vi "adam-4xxxl.vi"() -> ()   [LabVIEW 2024]
panel:
  in  "clear-command":bool
  in  "Channels":T1
  out "concatenated string":string
  in  "Single/Multi Channel":bool
  in  "Deliminator Char":string(combo)
  in  "Manual Command":string="#01"
  out "read buffer":string
  out "Bytes at Port":u32
  in  "send-command":bool
  out "Channel Number":string
  out "Channel State String":string
  out "Device Address":string
  in  "Device Address":i32=1 min=0 max=100 step=1
  in  "baud rate (19200)":u32=19200
  in  "COM Port (COM10)":refnum<visa-resource-name>="COM10"
  in  "Stop Program":bool
  out "command":string
  in  "Channel Number":i32=1 min=0 max=7 step=1
  in  "Channel State Bit":bool
  out "Bytes Written":u32
  out "error":errorcluster
  # "ADAM-4xxx Test VI"
  # "To Use, either:\n- Enter Manual Command in Text box\nOR\n- Set up command using options below\nThen:\n- Press Send Command"
  # "Example Commands:\n  Code   |    Behaviour       | Success | Failed \n---      |---                 |---      |---\nadam-4069 8x Power Relay\n#010000 \t| All Channels: Off  |\t   > \t  | ?AA \n#01000F \t| All Channels: On \t |         |\n#011000 \t| Channel 0: Off \t   |\t        |\n#011001 \t| Channel 0: On \t\t   |         |\n#011100 \t| Channel 1: Off \t\t  |         |\n#011101 \t| Channel 1: On \t    |         |"
  # "adam-4017+ 8x AI\nadam-4018+ 8x T/C & mA\n#01 \t    | All Channels: data |>+data+data...| ?AA \nAA = module address"
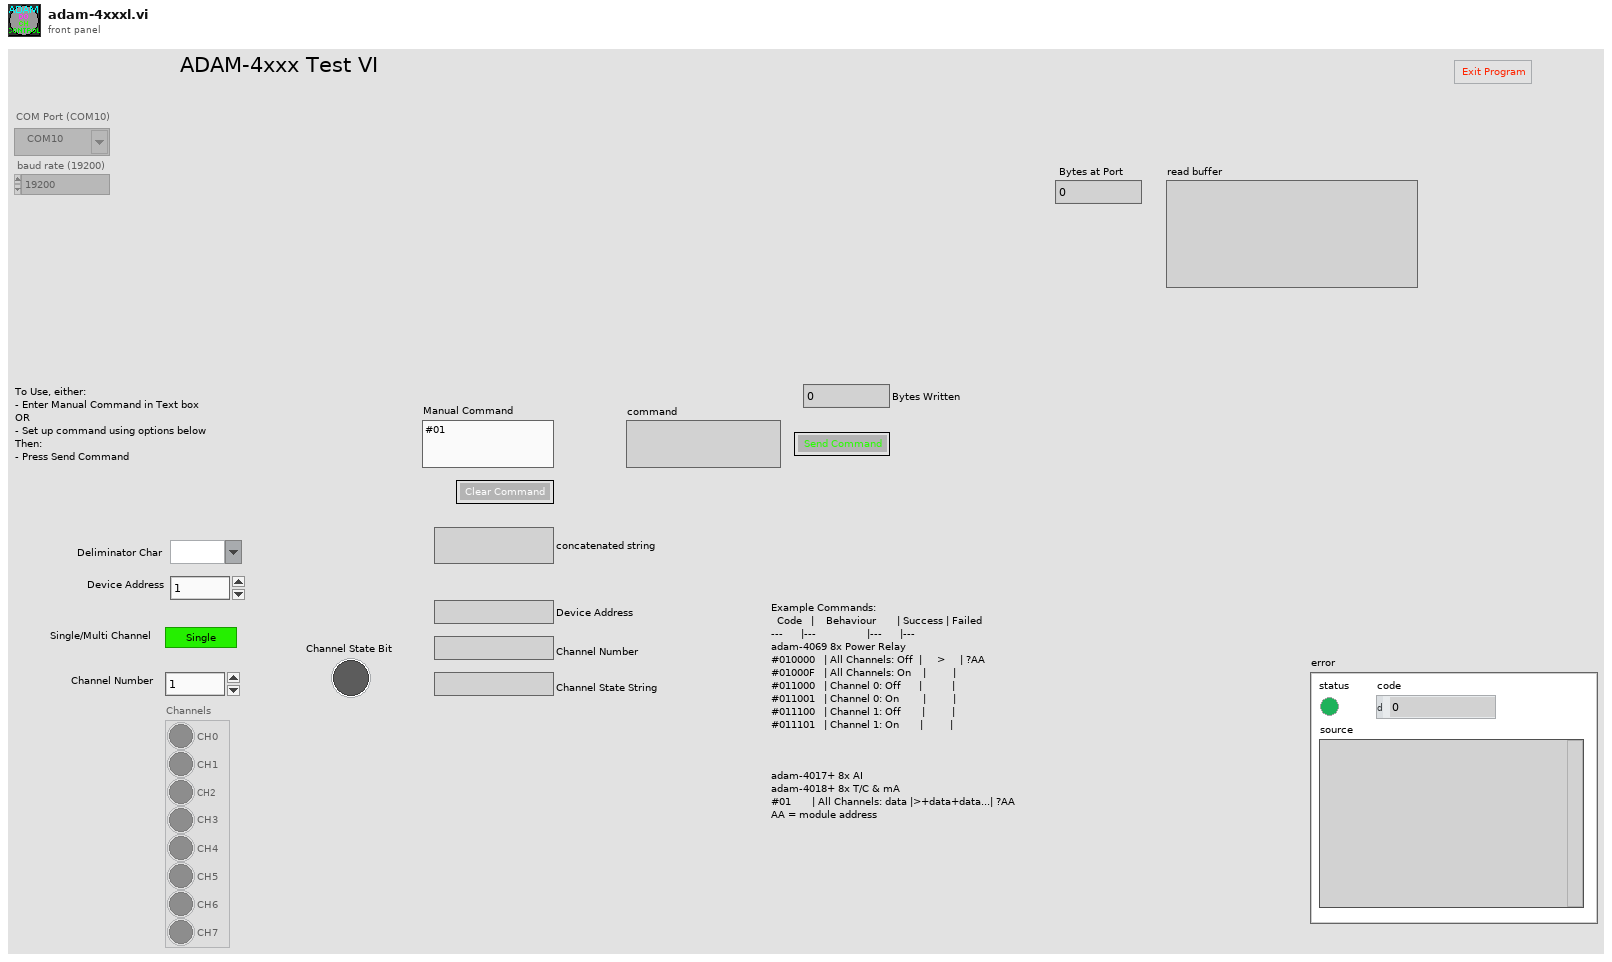
[diagram p1: front panel]
types:
  T1 = cluster{"CH0":bool, "CH1":bool, "CH2":bool, "CH3":bool, "CH4":bool, "CH5":bool, "CH6":bool, "CH7":bool}
  T2 = enum8{"Enabled", "Disabled", "Disabled and Grayed Out"}
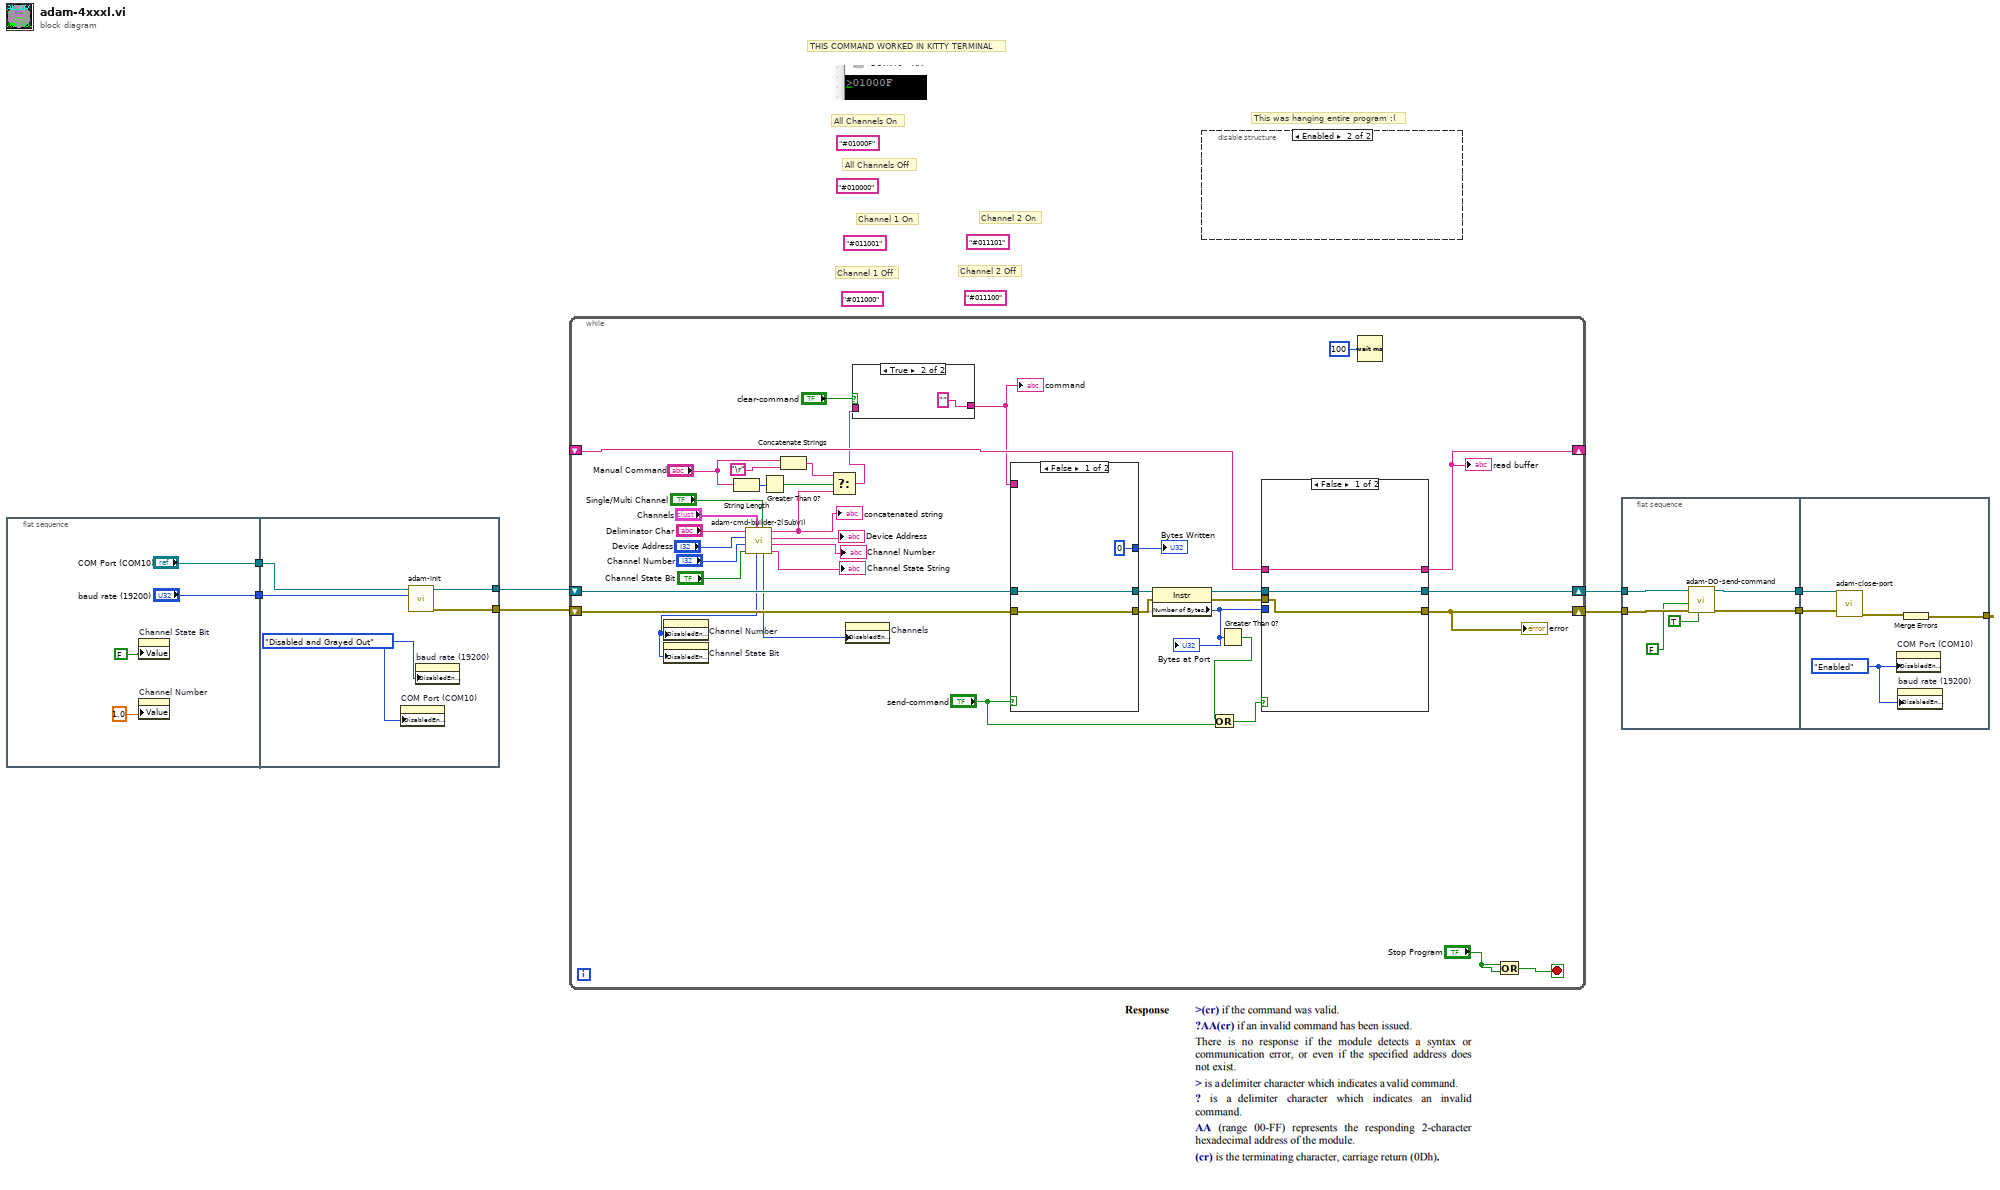
[diagram p0: block diagram]
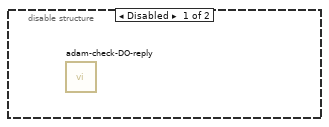
[diagram p2: hidden frame]
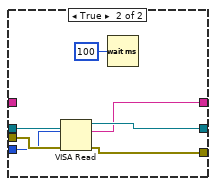
[diagram p4: hidden frame]
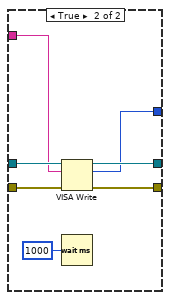
[diagram p5: hidden frame]
diagram:
  (unwired) "#011101" ("write buffer")
  (unwired) "#011100" ("write buffer")
  (unwired) "#011001" ("write buffer")
  (unwired) "#011000" ("write buffer")
  (unwired) "#010000" ("write buffer")
  (unwired) "#01000F" ("write buffer")
  # "This was hanging entire program :("
  # "Channel 2 Off"
  # "Channel 2 On"
  # "Channel 1 Off"
  # "Channel 1 On"
  # "All Channels Off"
  # "All Channels On"
  # "THIS COMMAND WORKED IN KITTY TERMINAL"
  n1 = flat-sequence {
    tunnel: ["baud rate (19200)"] -> w2
    tunnel: ["COM Port (COM10)"] -> w1
    tunnel: [w17] -> w6
    tunnel: [w16] -> w5
    tunnel: w2 -> [w15]
    tunnel: w1 -> [w14]
    frame #0 {
      n2 = property on="Channel State Bit" class="Bool (strict)"("Value"=FALSE ("Channel Active")) -> ()  [unwired: 2 in, 2 out]
      n3 = property on="Channel Number" class="DigNum (strict)"("Value"=1.0 ("Channel Number")) -> ()  [unwired: 2 in, 2 out]
    }
    frame #1 {
      w13 = T2."Disabled and Grayed Out" ("Disabled")
      n4 = property on="COM Port (COM10)" class="VISAName"("DisabledEnum"=w13) -> ()  [unwired: 2 in, 2 out]
      n5 = call "adam-init.vi"("baud rate (19200)"=w15, "COM Port (COM10)"=w14) -> ("error out"=w16:errorcluster, "VISA resource name out"=w17:refnum<visa-resource-name>)  [unwired: 8 in]
      n6 = property on="baud rate (19200)" class="DigNum (strict)"("DisabledEnum"=w13) -> ()  [unwired: 2 in, 2 out]
    }
  }
  n7 = while {
    shift-right: [w44] -> w7
    shift-left: w6 -> [w53]
    shift-right: [w27] -> w8
    shift-left: w5 -> [w52]
    shift-right: [w43] -> _
    shift-left: _ -> [w42]
    stop <- w55 stop-if-true
    n8 = String Length(string="Manual Command") -> (length=w41:i32)
    n9 = call "adam-cmd-builder-2(SubVI).vi"("Single/Multi Channel"="Single/Multi Channel", "Channels"="Channels", "Channel State Bit"="Channel State Bit", "Channel Number in"="Channel Number", "Device Address in"="Device Address", "Deliminator Char"="Deliminator Char") -> ("Channel State String"=→"Channel State String":string, "Channel Number out"=→"Channel Number":string, "Device Address out"=→"Device Address":string, "concatenated string"=w31:string, "MultiCH-enable"=w32:T2, "SingleCH-enable"=w33:T2)
    "concatenated string" <- w31
    n10 = property on="Channel Number" class="DigNum (strict)"("DisabledEnum"=w33) -> ()  [unwired: 2 in, 2 out]
    n11 = property on="Channel State Bit" class="Bool (strict)"("DisabledEnum"=w33) -> ()  [unwired: 2 in, 2 out]
    n12 = Greater Than 0?(x=w41) -> (x > 0?=w40:bool)
    n13 = Concatenate Strings("Manual Command", "\r") -> (w22:string)
    n14 = Select(t=w22, s=w40, f=w31) -> (s? t:f=w19:string)
    n15 = property on="Channels" class="Clust (strict)"("DisabledEnum"=w32) -> ()  [unwired: 2 in, 2 out]
    n16 = case shown="True" "clear-command" {
      tunnel: w19 -> [w56 _]
      tunnel: [w56 ""] -> w18
      frame False {
      }
      frame True {
      }
    }
    "command" <- w18
    n17 = case shown="False" "send-command" {
      tunnel: w53 -> [w69 w77]
      tunnel: w52 -> [w68 w76]
      tunnel: [w68 w75] -> w48
      tunnel: [w69 w74] -> w49
      tunnel: [u32 0 ("return count") w73] -> w51
      tunnel: w18 -> [_ w72]
      frame False {
      }
      frame True {
        n18 = VISA Write(VISA resource name=w77, write buffer=w72, error in (no error)=w76) -> (VISA resource name out=w74:refnum<visa-resource-name>, return count=w73:u32, error out=w75:errorcluster)
        n19 = Wait (ms)(milliseconds to wait=u32 1000) -> ()  [unwired: 1 out]
      }
    }
    "Bytes Written" <- w51
    n20 = property class="Instr"(reference=w49, error in=w48) -> (reference out=w46:refnum<visa-resource-name>, error out=w47:errorcluster, "Serial Settings:Number of Bytes at Serial Port"=w45:u32)
    "Bytes at Port" <- w45
    n21 = Greater Than 0?(x=w45) -> (x > 0?=w26:bool)
    n22 = Or(x=w26, y="send-command") -> (x .or. y?=w24:bool)
    n23 = case shown="False" w24 {
      tunnel: w47 -> [w59 w66]
      tunnel: w46 -> [w60 w67]
      tunnel: w45 -> [_ w65]
      tunnel: [w60 w64] -> w44
      tunnel: [w59 w63] -> w27
      tunnel: [w58 w62] -> w43
      tunnel: w42 -> [w58 _]
      frame False {
      }
      frame True {
        n24 = VISA Read(VISA resource name=w67, byte count=w65, error in (no error)=w66) -> (VISA resource name out=w64:refnum<visa-resource-name>, read buffer=w62:string, error out=w63:errorcluster)  [unwired: 1 out]
        n25 = Wait (ms)(milliseconds to wait=u32 100) -> ()  [unwired: 1 out]
      }
    }
    "read buffer" <- w43
    "error" <- w27
    n26 = Wait (ms)(milliseconds to wait=u32 100) -> ()  [unwired: 1 out]
    n27 = Or(x="Stop Program", y="Stop Program") -> (x .or. y?=w55:bool)
  }
  n28 = disable-structure shown="Enabled" {
    frame Disabled {
      n29 = call "adam-check-DO-reply.vi"() -> ()  [unwired: 7 in, 5 out]
    }
    frame Enabled {
    }
  }
  n30 = flat-sequence {
    tunnel: w8 -> [w83]
    tunnel: w7 -> [w79]
    tunnel: [w82] -> w4
    tunnel: [w80] -> w3
    tunnel: w4 -> [w86]
    tunnel: w3 -> [w87]
    tunnel: [w85] -> _
    frame #0 {
      n31 = call "adam-DO-send-command.vi"("Stop All"=TRUE, "error in (no error)"=w83, "Channel Active"=FALSE, "VISA Refnum in"=w79) -> ("error out"=w80:errorcluster, "VISA Refnum out"=w82:refnum<visa-resource-name>)  [unwired: 2 in, 4 out]
    }
    frame #1 {
      w84 = T2."Enabled" ("Disabled")
      n32 = call "adam-close-port.vi"("error in (no error)"=w87, "VISA Refnum in"=w86) -> ("error out"=w88:errorcluster)  [unwired: 9 in]
      n33 = property on="COM Port (COM10)" class="VISAName"("DisabledEnum"=w84) -> ()  [unwired: 2 in, 2 out]
      n34 = property on="baud rate (19200)" class="DigNum (strict)"("DisabledEnum"=w84) -> ()  [unwired: 2 in, 2 out]
      n35 = Merge Errors(w88) -> (w85:errorcluster)
    }
  }
